vi "CheckSpectrumFAT.vi"(8 "error in":errorcluster, 10 "FAT Settings":T1 {"Step Width" format="%#.3g"}, 11 "connection ID in":refnum<k5>) -> (0 "error out":errorcluster, 1 "Error Info":T3, 2 "OK":bool, 3 "connection ID out":refnum<k5>, 4 "Log String":string, 5 "Checked Spectrum Parameters":T2 {"Step Width" format="%#.3g"})   [LabVIEW 2015, in "ProdigyRemoteControl.lvlib"]
uses:
  ProdigyRemoteControl.lvlib
  DEFINITIONS/DEF_RcError.ctl
  DEFINITIONS/DEF_ValSpectrParas.ctl
  DEFINITIONS/DEF_FAT_Settings.ctl
  DEFINITIONS/DEF_RcCmd.ctl
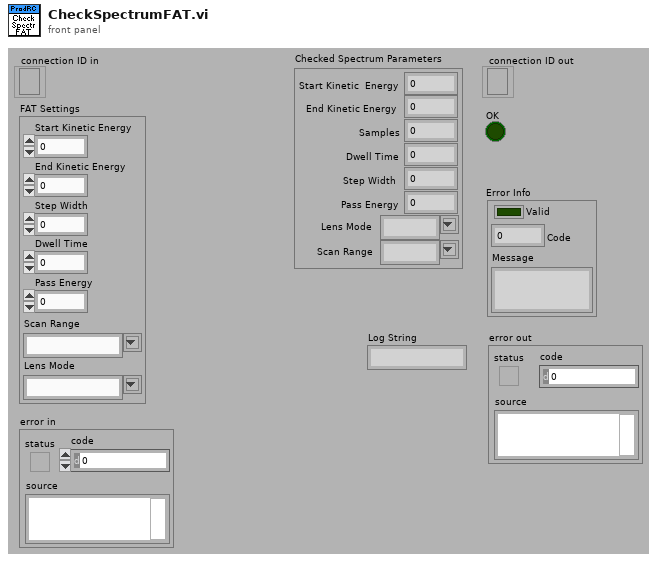
[diagram p1: front panel]
types:
  T1 = typedef "ProdigyRemoteControl.lvlib/DEF_FAT_Settings.ctl" = cluster{"Start Kinetic Energy":dbl, "End Kinetic Energy":dbl, "Step Width":dbl, "Dwell Time":dbl, "Pass Energy":dbl, "Scan Range":string, "Lens Mode":string}
  T2 = typedef "ProdigyRemoteControl.lvlib/DEF_ValSpectrParas.ctl" = cluster{"Start Kinetic  Energy":dbl, "End Kinetic Energy":dbl, "Samples":u32, "Dwell Time":dbl, "Step Width":dbl, "Pass Energy":dbl, "Lens Mode":string, "Scan Range":string}
  T3 = typedef "ProdigyRemoteControl.lvlib/DEF_RcError.ctl" = cluster{"Valid":bool, "Code":u16, "Message":string}
  T4 = typedef "ProdigyRemoteControl.lvlib/DEF_RcCmd.ctl" = string
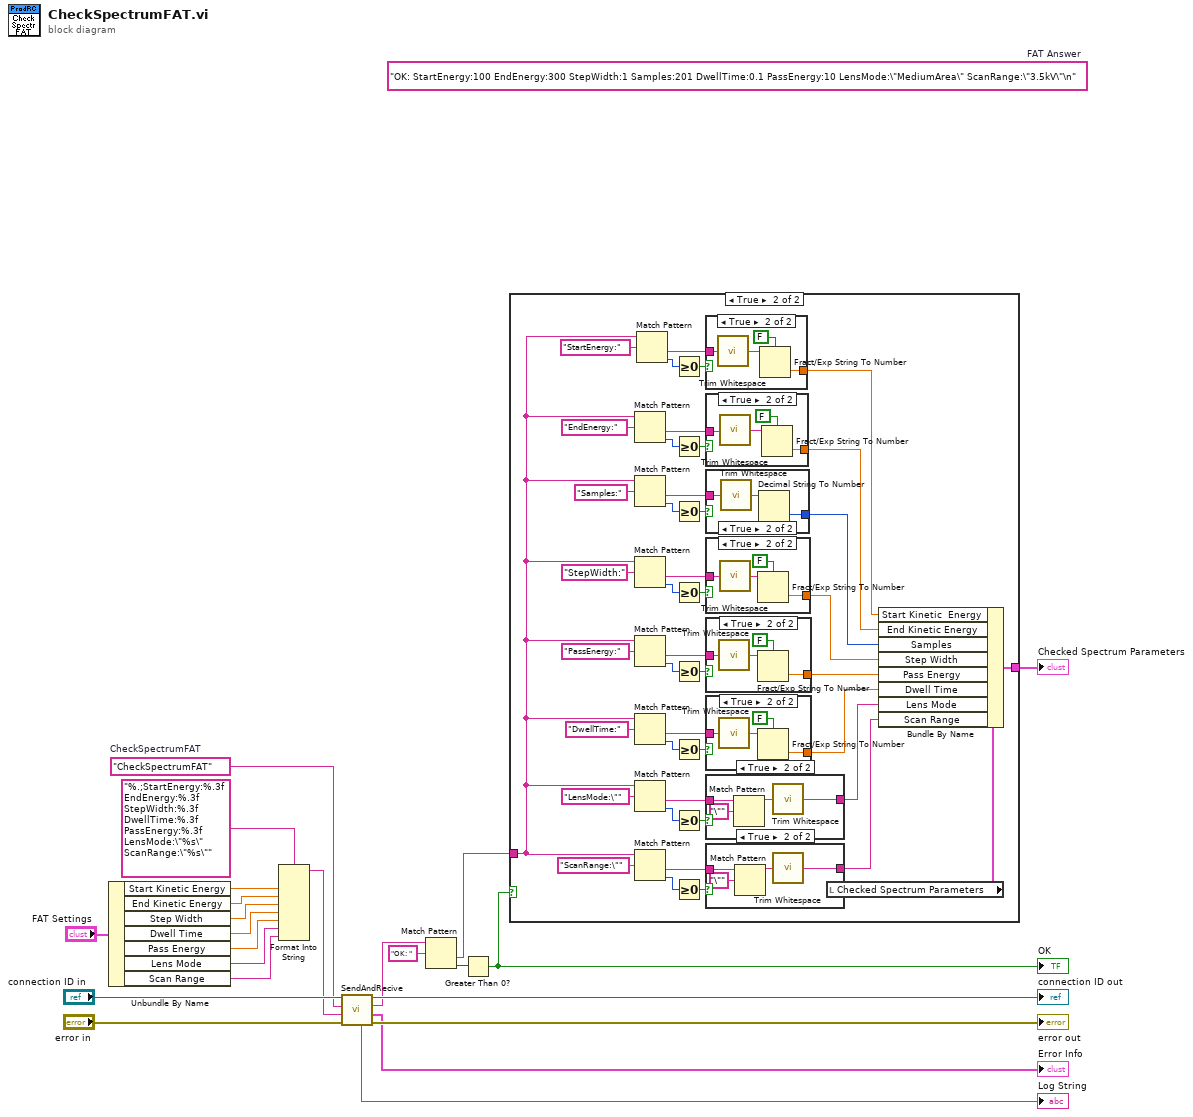
[diagram p0: block diagram]
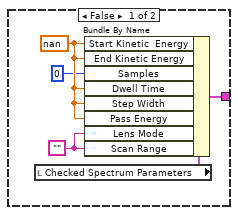
[diagram p2: hidden frame]
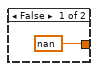
[diagram p3: hidden frame]
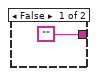
[diagram p4: hidden frame]
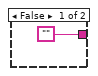
[diagram p5: hidden frame]
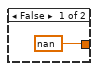
[diagram p6: hidden frame]
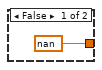
[diagram p7: hidden frame]
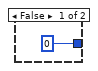
[diagram p8: hidden frame]
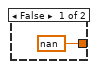
[diagram p9: hidden frame]
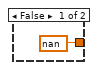
[diagram p10: hidden frame]
diagram:
  (unwired) "OK: StartEnergy:100 EndEnergy:300 StepWidth:1 Samples:201 DwellTime:0.1 PassEnergy:10 LensMode:\"MediumArea\" ScanRange:\"3.5kV\"\n"  # FAT Answer
  w3 = T4 "CheckSpectrumFAT"  # CheckSpectrumFAT
  n1 = Unbundle By Name("FAT Settings") -> ("Start Kinetic Energy"=w5:dbl, "End Kinetic Energy"=w6:dbl, "Step Width"=w7:dbl, "Dwell Time"=w8:dbl, "Pass Energy"=w9:dbl, "Lens Mode"=w10:string, "Scan Range"=w11:string)
  n2 = Format Into String(format string="%.;StartEnergy:%.3f EndEnergy:%.3f StepWidth:%.3f DwellTime:%.3f PassEnergy:%.3f LensMode:\"%s\" ScanRange:\"%s\"", w5, w6, w7, w8, w9, w10, w11) -> (resulting string=w2:string)  [unwired: 2 in, 1 out]
  n3 = call "SendAndRecive.vi"("error in"="error in", "Parameters"=w2, "Command"=w3, "connection ID in"="connection ID in") -> ("error out"=→"error out":errorcluster, "Error Info"=→"Error Info":T3, "Answer"=w17:string, "connection ID out"=→"connection ID out":refnum<k5>, "Log String"=→"Log String":string)  [unwired: 3 in]
  n4 = Match Pattern(string=w17, regular expression="OK: ") -> (after substring=w13:string, offset past match=w15:i32)  [unwired: 1 in, 2 out]
  n5 = Greater Than 0?(x=w15) -> (x > 0?=w12:bool)
  "OK" <- w12
  n6 = case shown="True" w12 {
    tunnel: w13 -> [_ w29]
    tunnel: [w27 w57] -> w14
    frame False {
      w24 = ""
      w26 = nan ("Start Kinetic  Energy")
      n7 = local read "Checked Spectrum Parameters"() -> (w28:T2)
      n8 = Bundle By Name(cluster=w28, "Start Kinetic  Energy"=w26, "End Kinetic Energy"=w26, "Samples"=u32 0, "Dwell Time"=w26, "Step Width"=w26, "Pass Energy"=w26, "Lens Mode"=w24, "Scan Range"=w24) -> (w27:T2)
    }
    frame True {
      n9 = Match Pattern(string=w29, regular expression="EndEnergy:") -> (after substring=w65:string, offset past match=w64:i32)  [unwired: 1 in, 2 out]
      n10 = Match Pattern(string=w29, regular expression="Samples:") -> (after substring=w62:string, offset past match=w61:i32)  [unwired: 1 in, 2 out]
      n11 = Match Pattern(string=w29, regular expression="StepWidth:") -> (after substring=w59:string, offset past match=w60:i32)  [unwired: 1 in, 2 out]
      n12 = Match Pattern(string=w29, regular expression="PassEnergy:") -> (after substring=w54:string, offset past match=w55:i32)  [unwired: 1 in, 2 out]
      n13 = Match Pattern(string=w29, regular expression="DwellTime:") -> (after substring=w35:string, offset past match=w34:i32)  [unwired: 1 in, 2 out]
      n14 = Match Pattern(string=w29, regular expression="LensMode:\"") -> (after substring=w49:string, offset past match=w48:i32)  [unwired: 1 in, 2 out]
      n15 = Match Pattern(string=w29, regular expression="ScanRange:\"") -> (after substring=w46:string, offset past match=w47:i32)  [unwired: 1 in, 2 out]
      n16 = Match Pattern(string=w29, regular expression="StartEnergy:") -> (after substring=w68:string, offset past match=w70:i32)  [unwired: 1 in, 2 out]
      n17 = Greater Or Equal To 0?(x=w70) -> (x >= 0?=w69:bool)
      n18 = Greater Or Equal To 0?(x=w64) -> (x >= 0?=w67:bool)
      n19 = Greater Or Equal To 0?(x=w61) -> (x >= 0?=w63:bool)
      n20 = Greater Or Equal To 0?(x=w60) -> (x >= 0?=w58:bool)
      n21 = Greater Or Equal To 0?(x=w55) -> (x >= 0?=w52:bool)
      n22 = Greater Or Equal To 0?(x=w34) -> (x >= 0?=w36:bool)
      n23 = Greater Or Equal To 0?(x=w48) -> (x >= 0?=w51:bool)
      n24 = Greater Or Equal To 0?(x=w47) -> (x >= 0?=w44:bool)
      n25 = case shown="True" w69 {
        tunnel: w68 -> [_ w110]
        tunnel: [nan w108] -> w43
        frame False {
        }
        frame True {
          n26 = call <vilib>:"Trim Whitespace.vi"("string"=w110) -> ("trimmed string"=w109:string)  [unwired: 1 in]
          n27 = Fract/Exp String To Number(use system decimal point (T)=FALSE, string=w109) -> (number=w108:dbl)  [unwired: 2 in, 1 out]
        }
      }
      n28 = case shown="True" w67 {
        tunnel: w65 -> [_ w105]
        tunnel: [nan w102] -> w42
        frame False {
        }
        frame True {
          n29 = call <vilib>:"Trim Whitespace.vi"("string"=w105) -> ("trimmed string"=w104:string)  [unwired: 1 in]
          n30 = Fract/Exp String To Number(use system decimal point (T)=FALSE, string=w104) -> (number=w102:dbl)  [unwired: 2 in, 1 out]
        }
      }
      n31 = case shown="True" w63 {
        tunnel: w62 -> [_ w100]
        tunnel: [0 w98] -> w40
        frame False {
        }
        frame True {
          n32 = call <vilib>:"Trim Whitespace.vi"("string"=w100) -> ("trimmed string"=w99:string)  [unwired: 1 in]
          n33 = Decimal String To Number(string=w99) -> (number=w98:i32)  [unwired: 2 in, 1 out]
        }
      }
      n34 = case shown="True" w58 {
        tunnel: w59 -> [_ w96]
        tunnel: [nan w93] -> w38
        frame False {
        }
        frame True {
          n35 = call <vilib>:"Trim Whitespace.vi"("string"=w96) -> ("trimmed string"=w94:string)  [unwired: 1 in]
          n36 = Fract/Exp String To Number(use system decimal point (T)=FALSE, string=w94) -> (number=w93:dbl)  [unwired: 2 in, 1 out]
        }
      }
      n37 = case shown="True" w52 {
        tunnel: w54 -> [_ w91]
        tunnel: [nan w88] -> w37
        frame False {
        }
        frame True {
          n38 = call <vilib>:"Trim Whitespace.vi"("string"=w91) -> ("trimmed string"=w89:string)  [unwired: 1 in]
          n39 = Fract/Exp String To Number(use system decimal point (T)=FALSE, string=w89) -> (number=w88:dbl)  [unwired: 2 in, 1 out]
        }
      }
      n40 = case shown="True" w36 {
        tunnel: w35 -> [_ w76]
        tunnel: [nan w73] -> w32
        frame False {
        }
        frame True {
          n41 = call <vilib>:"Trim Whitespace.vi"("string"=w76) -> ("trimmed string"=w74:string)  [unwired: 1 in]
          n42 = Fract/Exp String To Number(use system decimal point (T)=FALSE, string=w74) -> (number=w73:dbl)  [unwired: 2 in, 1 out]
        }
      }
      n43 = case shown="True" w51 {
        tunnel: w49 -> [_ w86]
        tunnel: ["" w85] -> w31
        frame False {
        }
        frame True {
          n44 = Match Pattern(string=w86, regular expression="\"") -> (before substring=w84:string)  [unwired: 1 in, 3 out]
          n45 = call <vilib>:"Trim Whitespace.vi"("string"=w84) -> ("trimmed string"=w85:string)  [unwired: 1 in]
        }
      }
      n46 = case shown="True" w44 {
        tunnel: w46 -> [_ w81]
        tunnel: ["" w80] -> w30
        frame False {
        }
        frame True {
          n47 = Match Pattern(string=w81, regular expression="\"") -> (before substring=w79:string)  [unwired: 1 in, 3 out]
          n48 = call <vilib>:"Trim Whitespace.vi"("string"=w79) -> ("trimmed string"=w80:string)  [unwired: 1 in]
        }
      }
      n49 = local read "Checked Spectrum Parameters"() -> (w56:T2)
      n50 = Bundle By Name(cluster=w56, "Start Kinetic  Energy"=w43, "End Kinetic Energy"=w42, "Samples"=w40, "Step Width"=w38, "Pass Energy"=w37, "Dwell Time"=w32, "Lens Mode"=w31, "Scan Range"=w30) -> (w57:T2)
    }
  }
  "Checked Spectrum Parameters" <- w14
